vi "name_file_gelain.vi"(3 "Identifier":string) -> (0 "appended path":path)   [LabVIEW 2025]
panel:
  in  "Connections":string
  in  "type":string
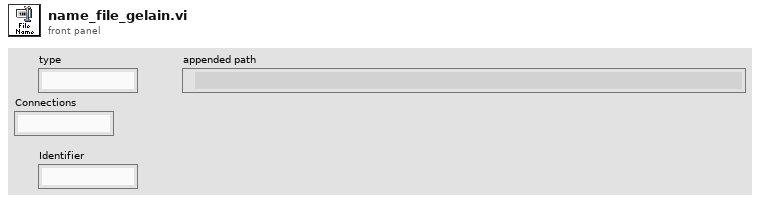
[diagram p1: front panel]
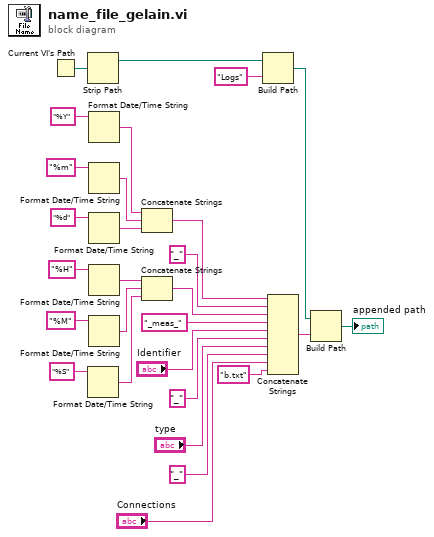
[diagram p0: block diagram]
diagram:
  n1 = Current VI's Path() -> (path=w25:path)
  n2 = Strip Path(path=w25) -> (stripped path=w1:path)  [unwired: 1 out]
  n3 = Format Date/Time String(time format string (%c)="%S") -> (date/time string=w16:string)  [unwired: 2 in]
  n4 = Format Date/Time String(time format string (%c)="%Y") -> (date/time string=w20:string)  [unwired: 2 in]
  n5 = Format Date/Time String(time format string (%c)="%m") -> (date/time string=w19:string)  [unwired: 2 in]
  n6 = Format Date/Time String(time format string (%c)="%d") -> (date/time string=w18:string)  [unwired: 2 in]
  n7 = Format Date/Time String(time format string (%c)="%H") -> (date/time string=w14:string)  [unwired: 2 in]
  n8 = Format Date/Time String(time format string (%c)="%M") -> (date/time string=w15:string)  [unwired: 2 in]
  n9 = Concatenate Strings(w20, w19, w18) -> (w17:string)
  n10 = Concatenate Strings(w14, w15, w16) -> (w9:string)
  n11 = Build Path(base path=w1, name or relative path="Logs") -> (appended path=w27:path)
  n12 = Concatenate Strings(w17, "_", w9, "_meas_" ("string"), "Identifier", "_", "type", "_", "Connections", "b.txt") -> (w24:string)
  n13 = Build Path(base path=w27, name or relative path=w24) -> (appended path=→"appended path":path)
